vi "hello.vi"(11 "input":string[](array[string])=[""]) -> (2 "output":string, 3 "return":i32)   [LabVIEW 2018]
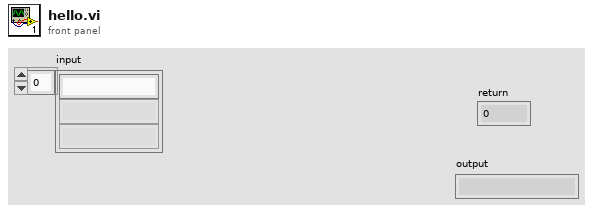
[diagram p1: front panel]
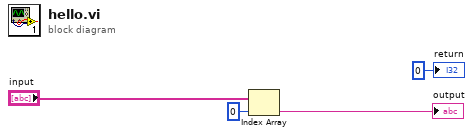
[diagram p0: block diagram]
diagram:
  n1 = Index Array(array="input", index=0) -> (element=→"output":string)
  "return" <- 0 ("return")
